vi "Interface_AddImplementVI.vi"(0 "Application":refnum<vi>, 1 "ClassRefToActOn":refnum<vi>, 2 "RefNameInClass":string, 3 "SubInterfaceImplementVI":path, 5 "error in":errorcluster) -> (19 "error out":errorcluster)   [LabVIEW 2012]
uses:
  <vilib>/Utility/miscctls.llb/LVPositionTypeDef.ctl
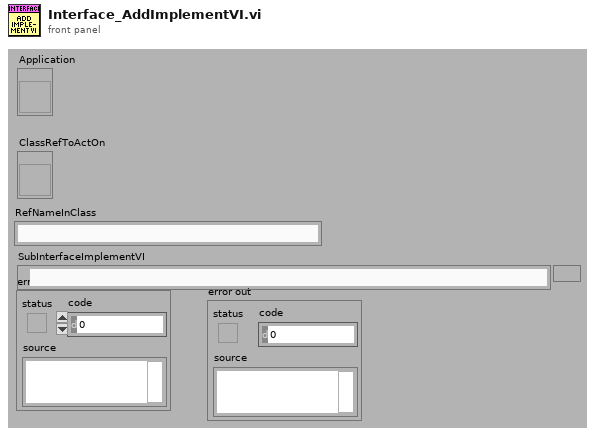
[diagram p1: front panel]
types:
  T1 = typedef "LVPositionTypeDef.ctl" = cluster{"Left":i32, "Top":i32}
  T2 = cluster{"IndTerm":refnum<vi>, "Bundler":refnum<vi>, "SourceTerm":refnum<vi>, "IndOwner":refnum<vi>, "IndPosition":T1, "ViRef":refnum<vi>, "Ind":refnum<vi>, "BundlerInTerm":refnum<vi>, "SourcePosition":T1, "BundlerIndex":i32}
  T3 = typedef "LVRectTypeDef.ctl" = cluster{"Left":i16, "Top":i16, "Right":i16, "Bottom":i16}
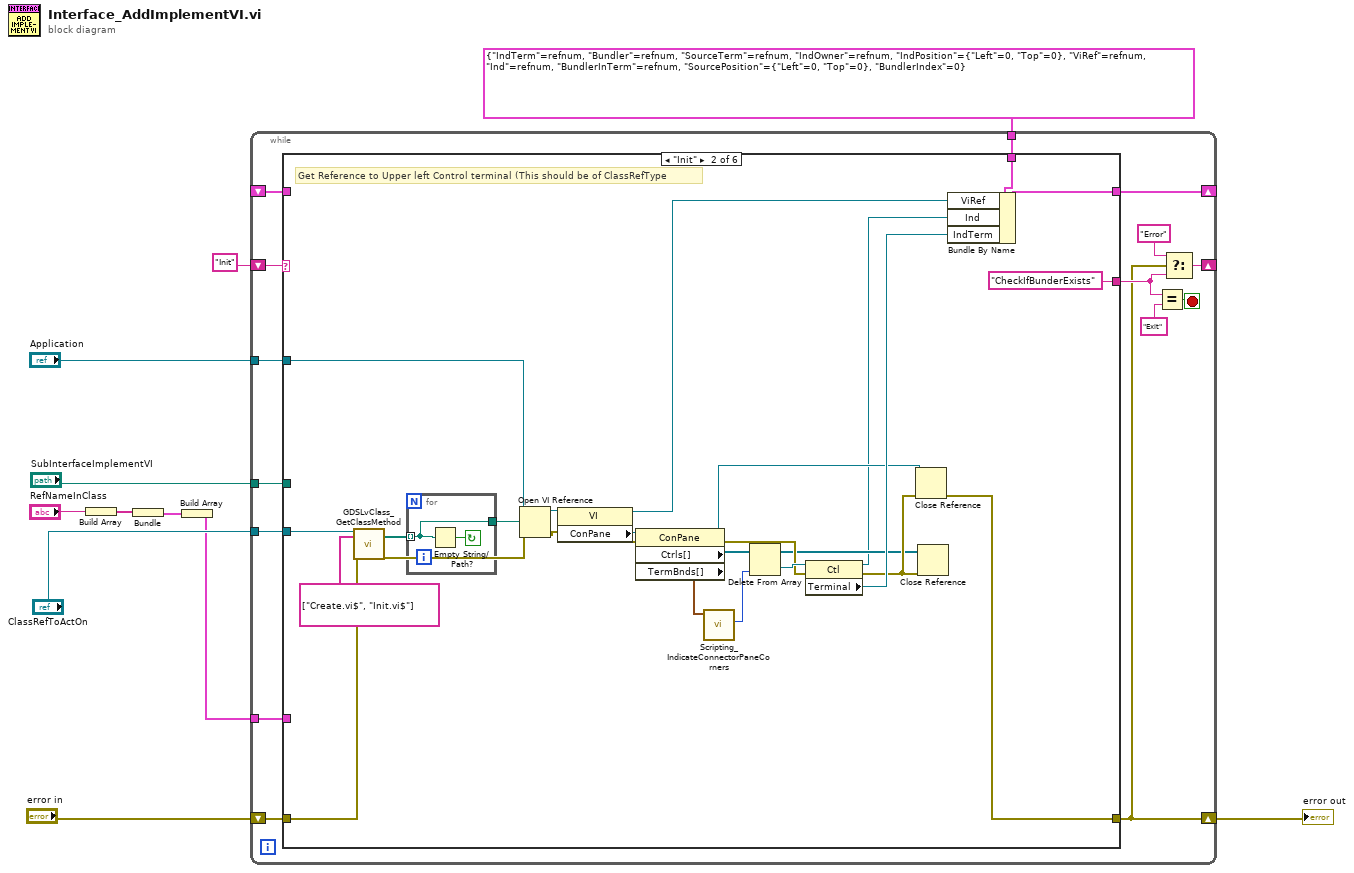
[diagram p0: block diagram]
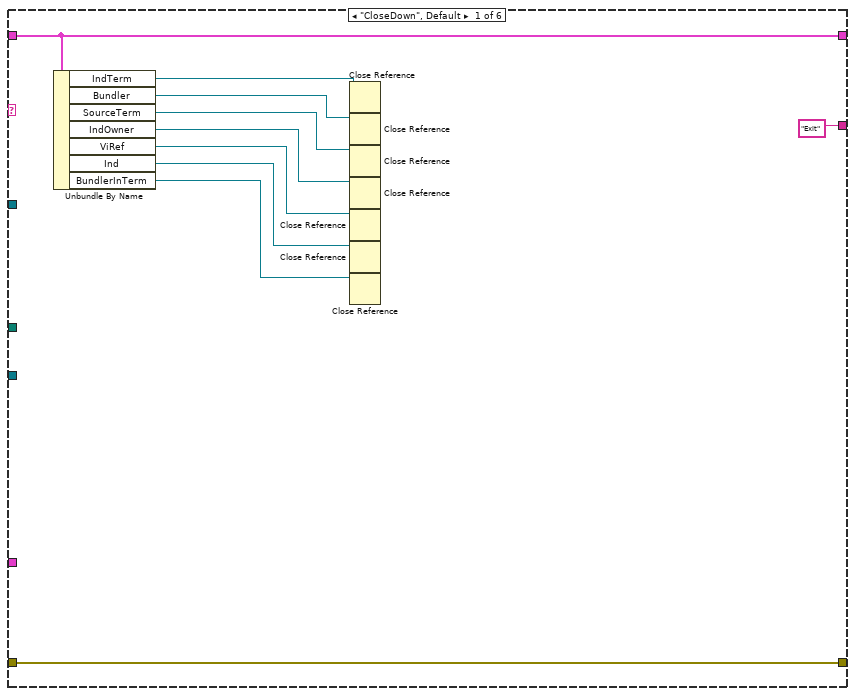
[diagram p2: hidden frame]
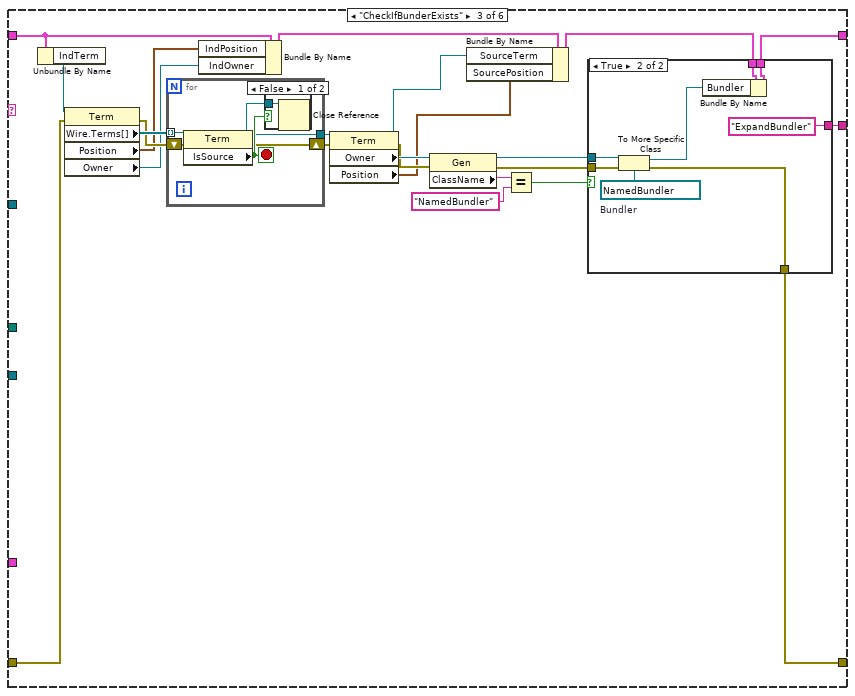
[diagram p3: hidden frame]
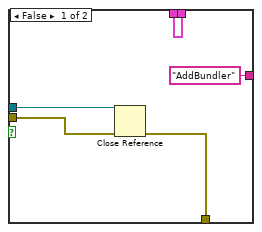
[diagram p4: hidden frame]
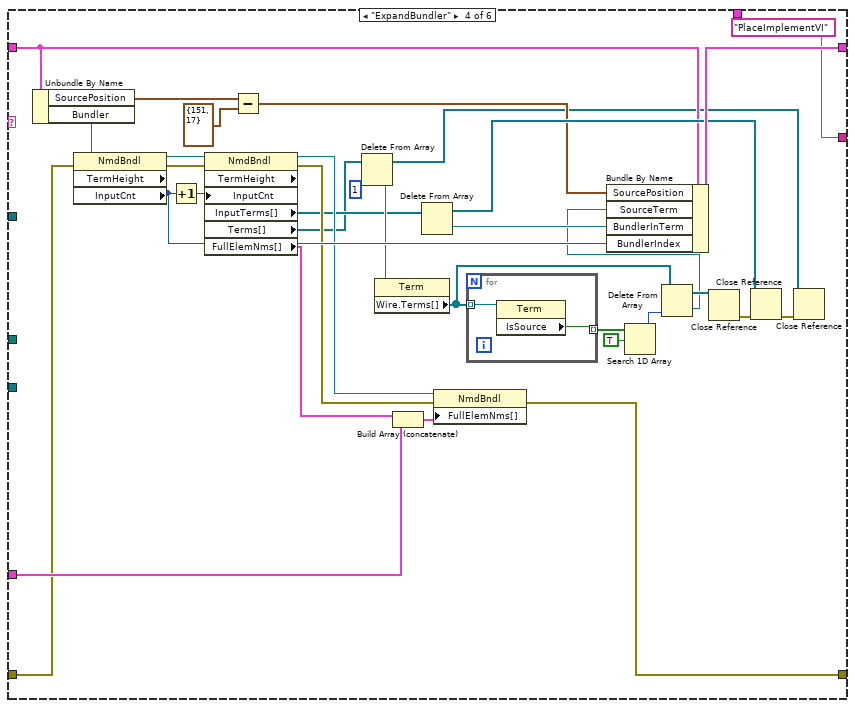
[diagram p6: hidden frame]
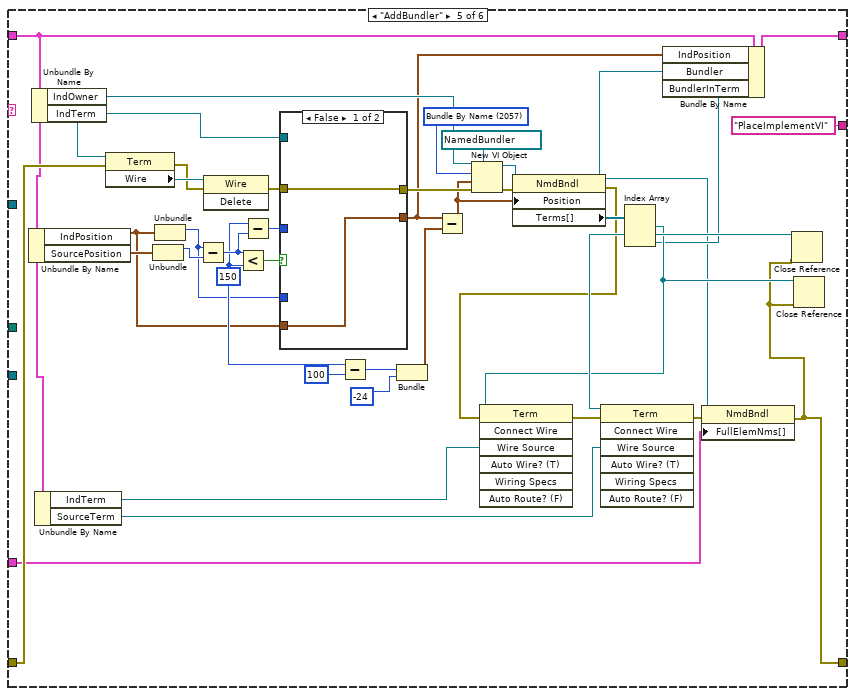
[diagram p7: hidden frame]
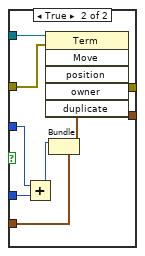
[diagram p8: hidden frame]
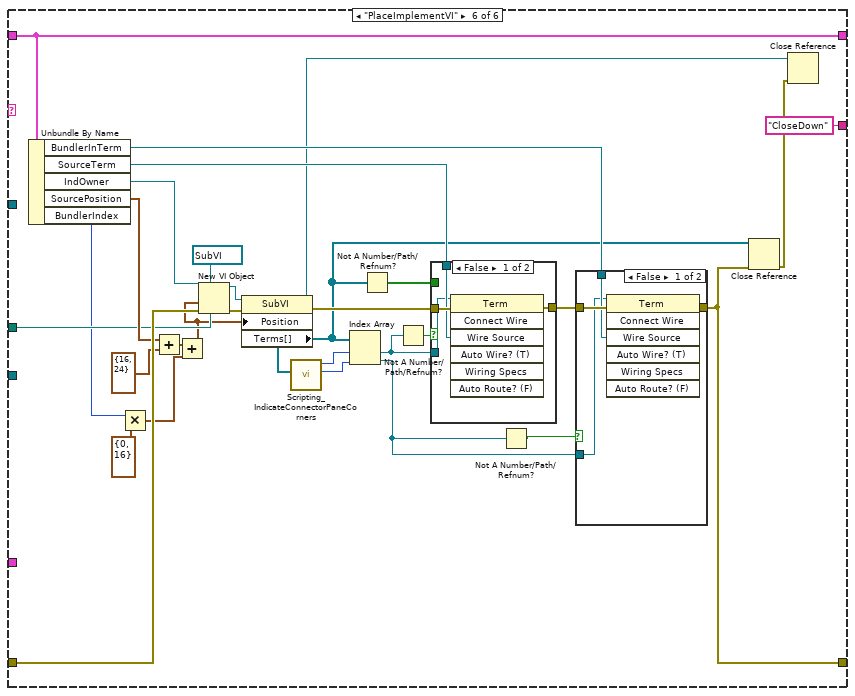
[diagram p9: hidden frame]
diagram:
  n1 = Build Array("RefNameInClass") -> (w4:string[])
  n2 = Bundle(w4) -> (w3:cluster{string[]})  [unwired: 1 in]
  n3 = Build Array(w3) -> (w2:cluster{string[]}[])
  n4 = while {
    shift-right: [w19] -> w8
    shift-left: "error in" -> [w26]
    shift-right: [w24] -> _
    shift-left: "Init" -> [w25]
    shift-right: [w18] -> _
    shift-left: _ -> [w17]
    tunnel: T2 {"IndTerm"=refnum, "Bundler"=refnum, "SourceTerm"=refnum, "IndOwner"=refnum, "IndPosition"={"Left"=0, "Top"=0}, "ViRef"=refnum, "Ind"=refnum, "BundlerInTerm"=refnum, "SourcePosition"={"Left"=0, "Top"=0}, "BundlerIndex"=0} -> [w16]
    tunnel: "ClassRefToActOn" -> [w15]
    tunnel: "Application" -> [w14]
    tunnel: w2 -> [w13]
    tunnel: "SubInterfaceImplementVI" -> [w12]
    stop <- w23 stop-if-true
    n5 = case shown="\"Init\"" w25 {
      tunnel: w26 -> [w36 w44 w70 w127 w179 w218]
      tunnel: [w36 w41 w69 w128 w146 w207] -> w19
      tunnel: ["Exit" "CheckIfBunderExists" w87 "PlaceImplementVI" "PlaceImplementVI" "CloseDown"] -> w20
      tunnel: [w34 w61 w80 w133 w160 w200] -> w18
      tunnel: w17 -> [w34 _ w73 w114 w157 w200]
      tunnel: w16 -> [_ w60 _ _ _ _]
      tunnel: w15 -> [_ w59 _ _ _ _]
      tunnel: w14 -> [_ w55 _ _ _ _]
      tunnel: w13 -> [_ _ _ w129 w145 _]
      tunnel: w12 -> [_ _ _ _ _ w214]
      frame "CloseDown", Default {
        n6 = Unbundle By Name(w34) -> ("IndTerm"=w33:refnum<vi>, "Bundler"=w32:refnum<vi>, "SourceTerm"=w31:refnum<vi>, "IndOwner"=w30:refnum<vi>, "ViRef"=w29:refnum<vi>, "Ind"=w28:refnum<vi>, "BundlerInTerm"=w27:refnum<vi>)
        n7 = Close Reference(reference=w33) -> ()  [unwired: 1 in, 1 out]
        n8 = Close Reference(reference=w32) -> ()  [unwired: 1 in, 1 out]
        n9 = Close Reference(reference=w31) -> ()  [unwired: 1 in, 1 out]
        n10 = Close Reference(reference=w30) -> ()  [unwired: 1 in, 1 out]
        n11 = Close Reference(reference=w29) -> ()  [unwired: 1 in, 1 out]
        n12 = Close Reference(reference=w28) -> ()  [unwired: 1 in, 1 out]
        n13 = Close Reference(reference=w27) -> ()  [unwired: 1 in, 1 out]
      }
      frame "Init" {
        # "Get Reference to Upper left Control terminal (This should be of ClassRefType"
        n14 = call <resource>:"GDSLvClass_GetClassMethod.vi"("Class Refnum In"=w59, "VINames"=string[] ["Create.vi$", "Init.vi$"], "error in (no error)"=w44) -> ("ViPaths"=w57:path[], "error out"=w54:errorcluster)  [unwired: 13 in, 2 out]
        n15 = for {
          tunnel: w57 -> [w63] mode=indexing
          tunnel: [w63] -> w56
          stop <- w64 continue-if-true
          n16 = Empty String/Path?(string/path=w63) -> (empty?=w64:bool)
        }
        n17 = Open VI Reference(application reference (local)=w55, vi path=w56, error in (no error)=w54) -> (vi reference=w53:refnum<vi>, error out=w49:errorcluster)  [unwired: 3 in]
        n18 = property class="VI"(reference=w53, error in=w49) -> (reference out=w43:refnum<vi>, error out=w50:errorcluster, "ConPane"=w52:refnum<vi>)
        n19 = property class="ConPane"(reference=w52, error in=w50) -> (reference out=w42:refnum<vi>, error out=w46:errorcluster, "Ctrls[]"=w45:refnum<vi>[], "TermBnds[]"=w51:T3[])
        n20 = call <resource>:"Scripting_IndicateConnectorPaneCorners.vi"("TermBnds[]"=w51) -> ("RightTop"=w37:i32)  [unwired: 7 in, 3 out]
        n21 = Delete From Array(array=w45, index=w37) -> (deleted portion=w48:refnum<vi>, array with subset deleted=w39:refnum<vi>[])  [unwired: 1 in]
        n22 = property class="Ctl"(reference=w48, error in=w46) -> (reference out=w38:refnum<vi>, error out=w40:errorcluster, "Terminal"=w47:refnum<vi>)
        n23 = Close Reference(reference=w42, error in (no error)=w40) -> (error out=w41:errorcluster)
        n24 = Close Reference(reference=w39, error in (no error)=w40) -> ()  [unwired: 1 out]
        n25 = Bundle By Name(cluster=w60, "ViRef"=w43, "Ind"=w38, "IndTerm"=w47) -> (w61:T2)
      }
      frame "CheckIfBunderExists" {
        n26 = Unbundle By Name(w73) -> ("IndTerm"=w86:refnum<vi>)
        n27 = property class="Term"(reference=w86, error in=w70) -> (error out=w74:errorcluster, "Wire.Terms[]"=w85:refnum<vi>[], "Position"=w72:T1, "Owner"=w71:refnum<vi>)  [unwired: 1 out]
        n28 = for {
          tunnel: w85 -> [w105] mode=indexing
          tunnel: [w103] -> w84
          shift-right: [w102] -> w75
          shift-left: w74 -> [w101]
          stop <- w104 stop-if-true
          n29 = property class="Term"(reference=w105, error in=w101) -> (reference out=w103:refnum<vi>, error out=w102:errorcluster, "IsSource"=w104:bool)
          n30 = case shown="False" w104 {
            tunnel: w103 -> [w106 _]
            frame False {
              n31 = Close Reference(reference=w106) -> ()  [unwired: 1 in, 1 out]
            }
            frame True {
            }
          }
        }
        n32 = Bundle By Name(cluster=w73, "IndPosition"=w72, "IndOwner"=w71) -> (w67:T2)
        n33 = property class="Term"(reference=w84, error in=w75) -> (reference out=w65:refnum<vi>, error out=w76:errorcluster, "Owner"=w83:refnum<vi>, "Position"=w68:T1)
        n34 = property class="Gen"(reference=w83, error in=w76) -> (reference out=w78:refnum<vi>, error out=w77:errorcluster, "ClassName"=w82:string)
        n35 = Bundle By Name(cluster=w67, "SourceTerm"=w65, "SourcePosition"=w68) -> (w66:T2)
        n36 = Equal?(x=w82, y="NamedBundler") -> (x = y?=w79:bool)
        n37 = case shown="True" w79 {
          tunnel: ["AddBundler" "ExpandBundler"] -> w87
          tunnel: w66 -> [w88 w99]
          tunnel: [w88 w98] -> w80
          tunnel: w78 -> [w92 w96]
          tunnel: w77 -> [w89 w95]
          tunnel: [w90 w93] -> w69
          frame False {
            n38 = Close Reference(reference=w92, error in (no error)=w89) -> (error out=w90:errorcluster)
          }
          frame True {
            w97 = refnum<vi> refnum  # Bundler
            n39 = To More Specific Class(target class=w97, reference=w96, error in=w95) -> (specific class reference=w94:refnum<vi>, error out=w93:errorcluster)
            n40 = Bundle By Name(cluster=w99, "Bundler"=w94) -> (w98:T2)
          }
        }
      }
      frame "ExpandBundler" {
        n41 = Unbundle By Name(w114) -> ("SourcePosition"=w113:T1, "Bundler"=w139:refnum<vi>)
        n42 = property class="NmdBndl" props=["TermHeight", "InputCnt"](reference=w139, error in=w127) -> (reference out=w138:refnum<vi>, error out=w137:errorcluster, "InputCnt"=w134:i32)  [unwired: 1 out]
        n43 = Increment(x=w134) -> (x+1=w136:i32)
        n44 = property class="NmdBndl" props=["TermHeight", "InputCnt", "InputTerms[]", "Terms[]", "FullElemNms[]"](reference=w138, error in=w137, "InputCnt"=w136) -> (reference out=w126:refnum<vi>, error out=w132:errorcluster, "InputTerms[]"=w110:refnum<vi>[], "Terms[]"=w109:refnum<vi>[], "FullElemNms[]"=w131:cluster{string[]}[])  [unwired: 1 out]
        n45 = Subtract(x=w113, y=T1 {"Left"=151, "Top"=17}) -> (x-y=w111:T1)
        n46 = Delete From Array(array=w109, index=1) -> (deleted portion=w124:refnum<vi>, array with subset deleted=w107:refnum<vi>[])  [unwired: 1 in]
        n47 = property class="Term"(reference=w124) -> ("Wire.Terms[]"=w121:refnum<vi>[])  [unwired: 1 in, 2 out]
        n48 = Build Array (concatenate)(w131, w129) -> (w130:cluster{string[]}[])
        n49 = Delete From Array(array=w110) -> (deleted portion=w135:refnum<vi>, array with subset deleted=w117:refnum<vi>[])  [unwired: 2 in]
        n50 = property class="NmdBndl"(reference=w126, error in=w132, "FullElemNms[]"=w130) -> (error out=w128:errorcluster)  [unwired: 1 out]
        n51 = for {
          tunnel: w121 -> [w141] mode=indexing
          tunnel: [w140] -> w123 mode=indexing
          n52 = property class="Term"(reference=w141) -> ("IsSource"=w140:bool)  [unwired: 1 in, 2 out]
        }
        n53 = Search 1D Array(1D array=w123, element=TRUE) -> (index of element=w120:i32)  [unwired: 1 in]
        n54 = Delete From Array(array=w121, index=w120) -> (deleted portion=w116:refnum<vi>, array with subset deleted=w119:refnum<vi>[])  [unwired: 1 in]
        n55 = Bundle By Name(cluster=w114, "SourcePosition"=w111, "SourceTerm"=w116, "BundlerInTerm"=w135, "BundlerIndex"=w134) -> (w133:T2)
        n56 = Close Reference(reference=w119) -> (error out=w118:errorcluster)  [unwired: 1 in]
        n57 = Close Reference(reference=w117, error in (no error)=w118) -> (error out=w108:errorcluster)
        n58 = Close Reference(reference=w107, error in (no error)=w108) -> ()  [unwired: 1 out]
      }
      frame "AddBundler" {
        w165 = 2057 items=[".NET Container"=2125, ".NET Refnum"=3441, "2D Picture"=3508, "3D Picture"=23776, "Absolute Value"=1054, "Access Rights"=1412, "ActiveX Container"=2072, "Add"=3915, "Add 1"=1050, "Add Array Elements"=1903, "Agitator"=3831, "AllSpoll"=1960, "Always Copy"=2400, "And"=1061, "And Array Elements"=1911, "Append True/False String"=1511, "Application Refnum"=3412, "Array"=21608, "Array 1"=3300, "Array Constant"=2070, "Array Interface Control"=23777, "Array Max & Min"=1907, "Array Size"=1809, "Array Subset"=2044, "Array To Cluster"=1168, "Array To Spreadsheet String"=1540, "Array of Strings to Path"=1422, "Atmospheric Tank"=3070, "Atmospheric Tank 1"=21751, "Automation Close"=8001, "Automation Open"=8000, "Automation Refnum"=3410, "Avogadro Constant (1/mol)"=23520, "Base 10 Logarithm Of e"=23512, "Bin"=3073, "Bin 1"=21755, "Bitpack to Array"=3135, "Blocking Variable Read"=23786, "Blocking Variable Write"=23789, "Bluetooth Close Connection"=9148, "Bluetooth Create Listener"=9151, "Bluetooth Discover"=9152, "Bluetooth Network Connection Refnum"=3468, "Bluetooth Open Connection"=9153, "Bluetooth Read"=9149, "Bluetooth Wait On Listener"=9147, "Bluetooth Write"=9150, "Boolean Array To Number"=1815, "Boolean To (0,1)"=1167, "Build Array"=2041, "Build Cluster Array"=2047, "Build Matrix"=8500, "Build Path"=1419, "Build Waveform"=2066, "Bundle"=2049, "Bundle By Name"=2057, "Byte Array To String"=1609, "Byte Stream File Refnum"=3408, "CAN Channel"=21966, "CAN Channel 1"=3340, "CAN Channel 2"=2124, "CAN Channel 3"=21817, "CAN Interface"=3339, "CAN Interface 1"=21815, "CAN Interface 2"=2123, "CAN Interface 3"=21964, "CAN Task"=3470, "CAN Task 1"=3471, "CAN Task 2"=21963, "CAN Task 3"=21789, "CPU Information"=24130, "Call By Reference Node"=3901, "Call Chain"=1999, "Call Library Function Node"=2062, "Call Parent Method"=2354, "Cancel Button"=21739, "Cancel Notification"=9107, "Carriage Return Constant"=23500, "Case Structure"=2001, "Cast Unit Bases"=1079, "Check Valve"=3833, "Checkbox"=3117, "Class Specifier Constant"=2094, "Classic Radio Buttons"=22003, "Clear Fixed-Point Overflow Status"=5562, "Close File"=1405, "Close File 1"=8052, "Close Reference"=8011, "Close Variable Connection"=23783, "Cluster"=3400, "Cluster 1"=21607, "Cluster Constant"=2071, "Cluster To Array"=1169, "Code Interface Node"=2050, "Coerce To Type"=2402, "Color Box"=3013, "Color Box Constant"=2120, "Color Box Thin Border"=2905, "Color Ramp"=3022, "Combo Box"=21604, "Combo Box 1"=3304, "Combo Box Constant"=2088, "Complex Conjugate"=1048, "Complex To Polar"=1045, "Complex To Re/Im"=1044, "Compound Arithmetic"=2200, "Compressor"=3832, "Concatenate Strings"=2040, "Conditional Disable Structure"=2064, "Constructor Node"=3904, "Control & Simulation Loop"=2099, "Control Help Window"=1353, "Control Online Help"=1355, "Control Refnum"=3419, "Convert Unit"=2059, "Conveyer"=3827, "Copy"=1416, "Copy 1"=8053, "Cosecant"=1204, "Cosine"=1201, "Cotangent"=1205, "Create Folder"=8055, "Create User Event"=2073, "Current Processor ID"=24131, "Current VI's Menubar"=9000, "Current VI's Path"=1426, "DAQmx Analog Trigger Source"=3336, "DAQmx Analog Trigger Source 1"=2119, "DAQmx Analog Trigger Source 2"=21951, "DAQmx Analog Trigger Source 3"=21774, "DAQmx Device Name"=21773, "DAQmx Device Name 1"=21950, "DAQmx Device Name 2"=2093, "DAQmx Device Name 3"=3318, "DAQmx Global Channel"=3443, "DAQmx Global Channel 1"=21770, "DAQmx Global Channel 2"=21957, "DAQmx Global Channel 3"=3430, "DAQmx Physical Channel"=3335, "DAQmx Physical Channel 1"=21954, "DAQmx Physical Channel 2"=2118, "DAQmx Physical Channel 3"=21777, "DAQmx Scale Name"=21952, "DAQmx Scale Name 1"=21775, "DAQmx Scale Name 2"=3317, "DAQmx Scale Name 3"=2116, "DAQmx Switch"=21953, "DAQmx Switch 1"=3337, "DAQmx Switch 2"=2121, "DAQmx Switch 3"=21776, "DAQmx Task Name"=3442, "DAQmx Task Name 1"=3434, "DAQmx Task Name 2"=21959, "DAQmx Task Name 3"=21778, "DAQmx Terminal"=21955, "DAQmx Terminal 1"=2117, "DAQmx Terminal 2"=21781, "DAQmx Terminal 3"=3319, "Data Cache Size"=24132, "Data Log File Refnum"=3402, "DataSocket Close"=1085, "DataSocket Open"=1084, "DataSocket Read"=1086, "DataSocket Refnum"=3417, "DataSocket Write"=1087, "Date/Time To Seconds"=1308, "Decimal Digit?"=1119, "Decimal String To Number"=1184, "Decimate 1D Array"=2046, "DecomposeArray"=2412, "DecomposeLockDataValRef"=2406, "DecomposeVariant"=2404, "Decrement"=1058, "Default Directory"=1427, "Delete"=8056, "Delete 1"=1417, "Delete Data Value Reference"=2409, "Delete From Array"=3912, "Delete Menu Items"=9004, "Delete Variant Attribute"=8206, "Delete Waveform Attribute"=8209, "Deny Access"=8057, "Dequeue Element"=9113, "Destroy User Event"=2075, "DevClear"=1961, "DevClearList"=1962, "Device Control/Status"=1433, "Device Refnum"=3405, "Diagram Disable Structure"=2054, "Dial"=3050, "Dial 1"=21732, "Digital Data"=3210, "Digital Data 1"=21216, "Digital Waveform Graph"=21718, "Digital Waveform Graph 1"=3511, "Direct Variable Read"=23785, "Direct Variable Write"=23788, "Divide"=1053, "Divide 1"=3918, "Dlg CheckBox"=21924, "Dlg Horiz Scrollbar"=21905, "Dlg Numeric"=2100, "Dlg Numeric 2"=3006, "Dlg String"=2110, "Dlg Vert Scrollbar"=21906, "Down Arrow"=3824, "Down Bow Valve"=3707, "Down Bow Valve 1"=21767, "Down Bow Valve 2"=3807, "Down Rect Valve"=21766, "Down Rect Valve 1"=3706, "Down Rect Valve 2"=3806, "Down Tee"=3818, "Down Tee 1"=3718, "EOF"=1410, "Elementary Charge (C)"=23517, "Empty Array?"=23063, "Empty Path Constant"=23523, "Empty String Constant"=23503, "Empty String/Path?"=1112, "Enable Menu Tracking"=9002, "EnableLocal"=1963, "EnableRemote"=1964, "End of Line Constant"=23525, "Enqueue Element"=9111, "Enqueue Element At Opposite End"=9129, "Enum"=3023, "Enum 1"=21605, "Enum Constant"=2090, "Equal To 0?"=1113, "Equal?"=1102, "Error Ring Constant"=2039, "Event Callback Refnum"=3435, "Event Data Node"=2102, "Event Structure"=2052, "Exchanger"=3828, "Exclusive Or"=1063, "Exponential"=1211, "Exponential (Arg) -1"=1222, "Expression Node"=2201, "FIFO Refnum"=3474, "False Constant"=2006, "Feedback Node, Feedback Node 1"=2353, "FieldPoint IO Point"=21784, "FieldPoint IO Point 1"=3440, "FieldPoint IO Point 2"=3439, "File Dialog"=8058, "File Dialog 1"=8081, "File Path Control"=21730, "File Path Control 1"=3203, "File Path Indicator"=21731, "File Path Indicator 1"=3204, "File/Directory Info"=1413, "File/Directory Info 1"=8082, "FindLstn"=1965, "FindRQS"=1966, "First Call?"=1083, "Fixed-Point Overflow?"=5565, "Fixed-Point to Integer Cast"=5566, "Flat Box"=3602, "Flat Circle"=3605, "Flat Down Triangle"=3623, "Flat Frame"=3608, "Flat Left Triangle"=3620, "Flat Right Triangle"=3621, "Flat Round Button"=3102, "Flat Rounded Box"=3611, "Flat Sequence Structure"=2069, "Flat Square Button"=3103, "Flat Up Triangle"=3622, "Flatten To String"=1164, "Flatten To XML"=8400, "Flattened String To Variant"=8202, "Floating Point Equal?"=23064, "Flush File"=8059, "Flush File 1"=1406, "Flush Queue"=9114, "For Loop"=2002, "Fork"=2194, "Format Date/Time String"=8100, "Format Into File"=2083, "Format Into String"=2081, "Format Value"=1512, "Formula Node"=2004, "Fract/Exp String To Number"=1187, "Framed Color Box"=21019, "Framed Color Box 1"=3008, "Free Label"=2321, "Furnace"=3829, "GPIB Clear"=1954, "GPIB Initialization"=1957, "GPIB Misc"=1956, "GPIB Read"=1951, "GPIB Serial Poll"=1955, "GPIB Status"=1959, "GPIB Trigger"=1953, "GPIB Wait"=1958, "GPIB Write"=1950, "Gauge"=21009, "Gauge 1"=3040, "Generate Front Panel Activity"=1329, "Generate Occurrence"=1700, "Generate User Event"=2074, "Generate User-Defined Trace Event"=2250, "Get Datalog Position"=8061, "Get Date/Time In Seconds"=1303, "Get Date/Time String"=1600, "Get Drag Drop Data"=9154, "Get File Position"=8062, "Get File Size"=8063, "Get Fixed-Point Components"=11163, "Get Help Window Status"=1354, "Get Matrix Diagonal"=8501, "Get Matrix Elements"=8502, "Get Menu Item Info"=9005, "Get Menu Selection"=9001, "Get Menu Short Cut Info"=9007, "Get Notifier Status"=9103, "Get Number of Records"=8064, "Get Permissions"=8065, "Get Queue Status"=9110, "Get Submatrix"=8503, "Get Type and Creator"=8066, "Get Variant Attribute"=8205, "Get Volume Info"=8067, "Get Waveform Attribute"=8208, "Get Waveform Components"=2067, "Global Variable"=2060, "Gravitational Constant (N m2/kg2)"=23519, "Greater Or Equal To 0?"=1114, "Greater Or Equal?"=1103, "Greater Than 0?"=1117, "Greater?"=1110, "Handle Peek"=1604, "Handle Poke"=1605, "Hex Digit?"=1123, "Hexadecimal String To Number"=1185, "Hopper"=21754, "Hopper 1"=3072, "Horiz Line"=3821, "Horiz Pipe"=3710, "Horiz Pipe 1"=3810, "Horizontal Button Box"=3636, "Horizontal Fill Slide"=3012, "Horizontal Fill Slide 1"=21100, "Horizontal Graduated Bar"=21106, "Horizontal Pointer Slide"=21101, "Horizontal Pointer Slide 1"=3011, "Horizontal Progress Bar"=21102, "Horizontal Scrollbar"=21110, "Horizontal Slide"=3010, "Horizontal Slide Switch"=3114, "Horizontal Smooth Box"=3633, "Horizontal Splitter Bar"=21861, "Horizontal Splitter Bar (Classic)"=21863, "Horizontal Splitter Bar (System)"=21865, "Horizontal Switch"=3108, "Horizontal Tank"=3071, "Horizontal Toggle Switch"=3110, "Horizontal Toggle Switch 1"=21700, "Hyperbolic Cosecant"=23053, "Hyperbolic Cosine"=1215, "Hyperbolic Cotangent"=23055, "Hyperbolic Secant"=23054, "Hyperbolic Sine"=1214, "Hyperbolic Tangent"=1216, "IMAQ Session"=3415, "IP To String"=1710, "IVI Delete Session"=8103, "IVI Logical Name"=3420, "IVI Logical Name 1"=3414, "IVI Logical Name 2"=21736, "IVI New Session"=8102, "Implies"=1080, "In Place Element Structure"=2360, "In Range and Coerce"=1127, "Include Fixed-Point Overflow Status"=5564, "Increment"=1057, "Index & Bundle Cluster Array"=2056, "Index Array"=2042, "Index String Array"=1531, "Initialize Array"=2053, "Inline C Node"=2104, "Insert Into Array"=3911, "Insert Menu Items"=9003, "Integer to Fixed-Point Cast"=5567, "Intensity Chart"=21719, "Intensity Chart 1"=3509, "Intensity Graph"=21720, "Intensity Graph 1"=3510, "Interleave 1D Arrays"=2045, "Interpolate 1D Array"=1905, "Inverse Cosecant"=23050, "Inverse Cosine"=1207, "Inverse Cotangent"=23052, "Inverse Hyperbolic Cosecant"=23056, "Inverse Hyperbolic Cosine"=1218, "Inverse Hyperbolic Cotangent"=23058, "Inverse Hyperbolic Secant"=23057, "Inverse Hyperbolic Sine"=1217, "Inverse Hyperbolic Tangent"=1219, "Inverse Secant"=23051, "Inverse Sine"=1206, "Inverse Tangent"=1208, "Inverse Tangent (2 Input)"=1228, "Invoke Node"=3900, "IrDA Close Connection"=9144, "IrDA Create Listener"=9140, "IrDA Discover"=9141, "IrDA Network Connection Refnum"=3450, "IrDA Open Connection"=9142, "IrDA Read"=9145, "IrDA Wait On Listener"=9143, "IrDA Write"=9146, "Join"=2195, "Join Numbers"=1171, "Junction"=2197, "Knob"=21000, "Knob 1"=3005, "LED Button"=3116, "LabVIEW Object"=3457, "Label"=21960, "Labeled Oblong Button"=3125, "Labeled Rectangular Button"=3124, "Labeled Round Button"=3122, "Labeled Square Button"=3123, "Leak Variant Value Reference"=2410, "Left Arrow"=3826, "Left Bow Valve"=3701, "Left Bow Valve 1"=3801, "Left Bow Valve 2"=21761, "Left Down Elbow"=3711, "Left Down Elbow 1"=3811, "Left Pump"=3713, "Left Pump 1"=3813, "Left Rect Valve"=3700, "Left Rect Valve 1"=21760, "Left Rect Valve 2"=3800, "Left Tee"=3709, "Left Tee 1"=3809, "Left Up Elbow"=3808, "Left Up Elbow 1"=3708, "Less Or Equal To 0?"=1115, "Less Or Equal?"=1104, "Less Than 0?"=1118, "Less?"=1111, "Lexical Class"=1126, "Line Feed Constant"=23501, "List Directory"=1418, "List Folder"=8083, "Listbox"=21792, "Listbox 1"=21806, "Listbox Symbol Ring Constant"=2038, "Local Variable"=2061, "Lock Range"=1411, "Logarithm Base 10"=1210, "Logarithm Base 2"=1225, "Logarithm Base X"=1224, "Logical Shift"=1081, "Lossy Enqueue Element"=9130, "Lowered Rounded Box"=3638, "MATLAB script"=9020, "Machine Epsilon"=23528, "MakeAddr"=1967, "Mantissa & Exponent"=1150, "Match First String"=1532, "Match Pattern"=1535, "Match True/False String"=1533, "MathScript Call By Reference Node"=3906, "MathScript Node"=2357, "Matrix Size"=8507, "Max & Min"=1108, "Menu Refnum"=3413, "Menu Ring"=3018, "Menu Ring 1"=21600, "Menu-Popup Ring"=3017, "Merge Signals"=2350, "Meter"=21008, "Meter 1"=3030, "Mixed Signal Graph"=21721, "Molar Gas Constant (J/(mol K))"=23522, "Motion Resource"=21787, "Motion Resource 1"=3448, "Motion Resource 2"=3449, "Motor"=3720, "Motor 1"=3820, "Move"=1415, "Move 1"=8068, "Multi-Segment Pipe"=23780, "Multicolumn Listbox"=21799, "Multicolumn Listbox 1"=21791, "Multiple Selection Listbox"=3208, "Multiply"=1052, "Multiply 1"=3917, "Multiply Array Elements"=1904, "Multirate Structure"=2199, "Natural Logarithm"=1209, "Natural Logarithm (Arg +1)"=1221, "Natural Logarithm Base"=23510, "Natural Logarithm Of 10"=23513, "Natural Logarithm Of 2"=23514, "Natural Logarithm Of Pi"=23508, "Negate"=1069, "Negative Infinity"=23509, "New Data Value Reference"=2408, "New Directory"=1402, "New File"=1404, "New VI"=8014, "New VI Object"=8015, "Not"=1064, "Not A Number/Path/Refnum?"=1128, "Not A Path Constant"=23524, "Not And"=1071, "Not Equal To 0?"=1116, "Not Equal?"=1105, "Not Exclusive Or"=1073, "Not Or"=1072, "Not a Refnum Constant"=23526, "Not a Shared Variable"=23527, "Notifier Refnum"=3423, "Number To Boolean Array"=1814, "Number To Decimal String"=1180, "Number To Engineering String"=1183, "Number To Exponential String"=1505, "Number To Fractional String"=1506, "Number To Hexadecimal String"=1181, "Number To Octal String"=1182, "Number of Cache Levels"=24133, "Numeric Constant"=2005, "Numeric Control"=3000, "Numeric Control 1"=21003, "Numeric Indicator"=3001, "Numeric Indicator 1"=21004, "OK Button"=21738, "OLE Variant"=3150, "Obtain Notifier"=9101, "Obtain Queue"=9108, "Occurrence Refnum"=3406, "Octal Digit?"=1129, "Octal String To Number"=1186, "Old VISA Open"=1921, "One Button Dialog"=1340, "Open Application Reference"=8012, "Open Device"=1430, "Open File"=1403, "Open Tank"=21752, "Open Tank 1"=3074, "Open VI Object Reference"=8013, "Open VI Reference"=8010, "Open Variable Connection"=23779, "Open Variable Connection in Background"=23791, "Open and Verify Variable Connection"=23790, "Open/Create/Replace Datalog"=8054, "Open/Create/Replace File"=8050, "Or"=1062, "Or Array Elements"=1910, "PPoll"=1969, "PPollConfig"=1970, "PPollUnconfig"=1971, "Package Matrix"=23001, "PassControl"=1968, "Path Constant"=2009, "Path To String"=1077, "Path Type"=1421, "Path to Array of Strings"=1423, "Pi"=23504, "Pi Divided By 2"=23506, "Pi Multiplied By 2"=23505, "Pick Line"=1510, "Pict Ring"=21602, "Pict Ring 1"=3015, "PixMap"=3505, "PixMap (Do not touch it!!)"=3507, "Planck's Constant (J/Hz)"=23516, "Platform Flat Square Button"=3134, "Plug-In Control"=21820, "Polar To Complex"=1047, "Polar To Re/Im"=23061, "Positive Infinity"=23515, "Power Of 10"=1212, "Power Of 2"=1223, "Power Of X"=1213, "Preserve Run-Time Class"=8018, "Pressure Tank"=3075, "Pressure Tank 1"=21753, "Preview Queue Element"=9112, "Printable?"=1124, "Property Node"=1920, "Pulldown Menu Ring"=3061, "Push Button"=21001, "Queue Refnum"=3424, "Quit LabVIEW"=1352, "Quotient & Remainder"=1056, "RT FIFO Create"=24000, "RT FIFO Delete"=24003, "RT FIFO Read"=24001, "RT FIFO Write"=24002, "Radio Buttons"=22001, "Raised Box"=3600, "Raised Box 1"=3637, "Raised Circle"=3603, "Raised Down Triangle"=3615, "Raised Frame"=3606, "Raised Left Triangle"=3612, "Raised Right Triangle"=3613, "Raised Rounded Box"=3609, "Raised Up Triangle"=3614, "Random Number (0-1)"=1070, "RcvRespMsg"=1972, "Re/Im To Complex"=1046, "Re/Im To Polar"=23060, "Read Datalog"=8069, "Read Device"=1432, "Read File"=1407, "Read Variable"=23781, "Read from Binary File"=8051, "Read from Text File"=8070, "ReadStatus"=1973, "Receive"=1974, "ReceiveSetup"=1975, "Recessed Box"=3601, "Recessed Circle"=3604, "Recessed Down Triangle"=3619, "Recessed Frame"=3607, "Recessed Left Triangle"=3616, "Recessed Menu Ring"=3019, "Recessed Right Triangle"=3617, "Recessed Rounded Box"=3610, "Recessed Up Triangle"=3618, "Reciprocal"=1059, "Reciprocal Of Pi"=23507, "Reciprocal Of e"=23511, "RecomposeArray"=2403, "RecomposeUnlockDataValRef"=2407, "RecomposeVariant"=2405, "Rectangular Stop Button"=3128, "Refnum to Path"=1424, "Refnum to Session"=2306, "Region"=2196, "Register Event Callback"=2078, "Register For Events"=2065, "Register Session"=2319, "Release Notifier"=9102, "Release Queue"=9109, "Remove Fixed-Point Overflow Status"=5563, "Replace Array Subset"=3910, "Replace Substring"=3913, "Request Deallocation"=1610, "ResetSys"=1976, "Reshape Array"=2055, "Resize Matrix"=8508, "Reverse 1D Array"=1900, "Reverse String"=1537, "Right Arrow"=3825, "Right Bow Valve"=21765, "Right Bow Valve 1"=3705, "Right Bow Valve 2"=3805, "Right Down Elbow"=3817, "Right Down Elbow 1"=3717, "Right Pump"=3719, "Right Pump 1"=3819, "Right Rect Valve"=3804, "Right Rect Valve 1"=3704, "Right Rect Valve 2"=21764, "Right Tee"=3715, "Right Tee 1"=3815, "Right Up Elbow"=3814, "Right Up Elbow 1"=3714, "Ring Constant"=2008, "Rocker"=21002, "Rotary Feeder"=3830, "Rotate"=1082, "Rotate 1D Array"=1906, "Rotate Left With Carry"=1606, "Rotate Right With Carry"=1607, "Rotate String"=1536, "Round Button"=3100, "Round LED"=3120, "Round LED 1"=21012, "Round Light"=3104, "Round Push Button"=3112, "Round Push Button 2"=3118, "Round Radio Button"=3106, "Round Stop Button"=3127, "Round To Nearest"=1055, "Round Toward +Infinity"=1076, "Round Toward -Infinity"=1075, "Rydberg Constant (1/m)"=23521, "Scale By Power Of 2"=1074, "Scan From File"=2082, "Scan From String"=2080, "Scan String For Tokens"=8101, "Scan Value"=1534, "Scanned Variable Read"=23784, "Scanned Variable Write"=23787, "Search 1D Array"=1901, "Search and Replace String"=3914, "Search/Split String"=1538, "Secant"=1203, "Seconds To Date/Time"=1309, "Seek"=1409, "Select"=1516, "Send"=1977, "Send Notification"=9104, "SendCmds"=1978, "SendDataBytes"=1979, "SendIFC"=1980, "SendLLO"=1982, "SendList"=1981, "SendSetup"=1983, "Session to Refnum"=2307, "Set Datalog Position"=8072, "Set File Position"=8073, "Set File Size"=8074, "Set Matrix Diagonal"=8504, "Set Matrix Elements"=8505, "Set Menu Item Info"=9006, "Set Number of Records"=8075, "Set Occurrence"=1702, "Set Permissions"=8076, "Set Submatrix"=8506, "Set Type and Creator"=8077, "Set Variant Attribute"=8204, "Set Waveform Attribute"=8207, "SetRWLS"=1984, "SetTimeOut"=1985, "Shared Variable"=23778, "Shared Variable Constant"=3473, "Shared Variable Control"=3472, "Shared Variable Control 1"=21814, "Shared Variable to String"=1831, "Sign"=1049, "Simple Horizontal Slide"=3003, "Simple Numeric"=3029, "Simple Numeric 1"=2900, "Simple String"=2115, "Simple Vertical Slide"=3002, "Sinc"=1227, "Sine"=1200, "Sine & Cosine"=1220, "Size Handle"=1603, "Slide Switch"=21011, "Sort 1D Array"=1120, "Sort Array of String, Sort Array of String 1"=23065, "Speed Of Light In Vacuum (m/sec)"=23518, "Split 1D Array"=1908, "Split Button"=21020, "Split Number"=1170, "Split Signals"=2351, "Spreadsheet String To Array"=1539, "Square"=23059, "Square Button"=3101, "Square LED"=3121, "Square LED 1"=21013, "Square Light"=3105, "Square Push Button"=3113, "Square Push Button 2"=3119, "Square Radio Button"=3107, "Square Root"=1060, "Stacked Sequence Structure"=2000, "State"=2198, "State Diagram"=2051, "Static VI Reference"=2084, "Stop"=1350, "Stop Button"=21230, "String Constant"=2007, "String Control"=3200, "String Control 1"=21701, "String Indicator"=3201, "String Indicator 1"=21702, "String Length"=1502, "String Subset"=1503, "String To Byte Array"=1608, "String To IP"=1711, "String To Path"=1078, "String to Shared Variable"=1830, "Strip Path"=1420, "SubPanel"=21810, "SubPanel (Classic)"=21811, "SubPanel (System)"=21823, "Subtract"=1051, "Subtract 1"=3916, "Swap Bytes"=1162, "Swap Values"=2401, "Swap Vector Element"=1912, "Swap Words"=1163, "System Button"=3130, "System Cancel Button"=3131, "System Checkbox"=3132, "System Chiseled Line"=3632, "System Colored Rectangle"=3625, "System Combo Box"=21917, "System Enum"=3062, "System Horizontal Pointer Slide"=21902, "System Horizontal Progress Bar"=21910, "System Horizontal Slide"=21904, "System Label"=21961, "System Listbox"=21805, "System Mixed Checkbox"=21333, "System Multicolumn Listbox"=21798, "System Numeric"=21919, "System Path Control"=21922, "System Pict Ring"=21925, "System Radio Button"=3133, "System Radio Buttons"=22002, "System Recessed Frame"=3624, "System Ring"=3060, "System Spin Control"=21900, "System String"=21920, "System Tab Control"=3331, "System Table"=21797, "System Time Stamp"=21967, "System Tree"=21794, "System Vertical Pointer Slide"=21901, "System Vertical Progress Bar"=21909, "System Vertical Slide"=21903, "TCP Close Connection"=1713, "TCP Create Listener"=1717, "TCP Flattened Read"=1718, "TCP Flattened Write"=1719, "TCP Flex Read"=1720, "TCP Flex Write"=1721, "TCP Network Connection Refnum"=3407, "TCP Open Connection"=1715, "TCP Read"=1716, "TCP Wait On Listener"=1712, "TCP Write"=1714, "TDMS Close"=24113, "TDMS Defragment"=24119, "TDMS File"=3477, "TDMS Flush"=24117, "TDMS Get Properties"=24115, "TDMS List Contents"=24116, "TDMS Open"=24112, "TDMS Read"=24111, "TDMS Refnum To File ID"=24120, "TDMS Set Properties"=24114, "TDMS Write"=24110, "TDMS Write IP"=24118, "Tab Constant"=23502, "Tab Control"=3330, "Tab Control 1"=3332, "Table"=21796, "Table 1"=21790, "Tag Attribute Ring"=2063, "Tangent"=1202, "Tank"=21006, "Tank 1"=3020, "Temporary Directory"=1435, "TestSRQ"=1986, "TestSys"=1987, "Text & Pict Ring"=21603, "Text & Pict Ring 1"=3016, "Text Button"=21015, "Text Ring"=21601, "Text Ring 1"=3014, "Text to UTF-8"=23066, "Thermometer"=21007, "Thermometer 1"=3021, "Thick Chiseled Line"=3630, "Thick Line"=3629, "Thick Line with Arrow"=3631, "Thick Lowered Box"=3635, "Thin Chiseled Line"=3627, "Thin Line"=3626, "Thin Line with Arrow"=3628, "Threshold 1D Array"=1909, "Tick Count (ms)"=1300, "Time Stamp Constant"=2068, "Time Stamp Control"=21913, "Time Stamp Control 1"=5555, "Time Stamp Indicator"=21914, "Time Stamp Indicator 1"=5556, "Timed Loop"=5570, "Timed Sequence"=5573, "To Byte Integer"=1140, "To Double Precision Complex"=1152, "To Double Precision Float"=1147, "To Extended Precision Complex"=1154, "To Extended Precision Float"=1149, "To Fixed-Point"=5561, "To Long Integer"=1142, "To Lower Case"=1189, "To More Generic Class"=8017, "To More Specific Class"=8016, "To OLE Variant"=8002, "To Probe String"=2413, "To Quad Integer"=1155, "To Single Precision Complex"=1151, "To Single Precision Float"=1146, "To Time Stamp"=5560, "To Unsigned Byte Integer"=1143, "To Unsigned Long Integer"=1145, "To Unsigned Quad Integer"=1156, "To Unsigned Word Integer"=1144, "To Upper Case"=1188, "To Variant"=8201, "To Word Integer"=1141, "Traditional DAQ Channel"=21733, "Traditional DAQ Channel 1"=2085, "Traditional DAQ Channel 2"=3320, "Transpose 1D Array"=23068, "Transpose 2D Array"=1902, "Transpose Matrix"=8509, "Tree"=21819, "Tree 1"=21793, "Trigger"=1988, "TriggerList"=1989, "Two Button Dialog"=1341, "Type Cast"=1166, "Type and Creator"=1434, "UDP Close"=1726, "UDP Multicast Open"=1727, "UDP Network Connection Refnum"=3418, "UDP Open"=1723, "UDP Read"=1724, "UDP Write"=1725, "UTF-8 to Text"=23067, "Unbitpack from Array"=3136, "Unbundle"=2048, "Unbundle By Name"=2058, "Unflatten From String"=1165, "Unflatten From XML"=8401, "Unleak Variant Value Reference"=2411, "Unpackage Matrix"=23000, "Unregister For Events"=2076, "Unregister Session"=2320, "Up Arrow"=3823, "Up Bow Valve"=3703, "Up Bow Valve 1"=3803, "Up Bow Valve 2"=21763, "Up Rect Valve"=3702, "Up Rect Valve 1"=21762, "Up Rect Valve 2"=3802, "Up Tee"=3712, "Up Tee 1"=3812, "User Defined Refnum"=3428, "User Defined Refnum Tag"=21745, "User Defined Refnum Tag 1"=3429, "User Defined Refnum Tag Constant"=3426, "User Defined Refnum Tag Flatten"=21747, "User Defined Refnum Tag Flatten 1"=3454, "User Defined Tag"=21749, "User Defined Tag 1"=3329, "User Defined Tag Constant"=2114, "User Item"=3506, "VI Library"=1425, "VI Refnum"=3422, "VI Server Reference"=2091, "VISA Assert Interrupt Signal"=2309, "VISA Assert Trigger"=1929, "VISA Assert Utility Signal"=2310, "VISA Clear"=1927, "VISA Close"=1922, "VISA Disable Event"=1940, "VISA Discard Events"=1941, "VISA Enable Event"=1942, "VISA Find Resource"=1923, "VISA Flush I/O Buffer"=2302, "VISA GPIB Command"=2315, "VISA GPIB Control ATN"=2316, "VISA GPIB Control REN"=2304, "VISA GPIB Pass Control"=2317, "VISA GPIB Send IFC"=2318, "VISA In 16"=1930, "VISA In 32"=1944, "VISA In 64"=2140, "VISA In 8"=1936, "VISA Lock"=1993, "VISA Map Address"=1932, "VISA Map Trigger"=2311, "VISA Memory Allocation"=1997, "VISA Memory Allocation Ex"=2146, "VISA Memory Free"=1998, "VISA Move"=2303, "VISA Move In 16"=1948, "VISA Move In 32"=1991, "VISA Move In 64"=2144, "VISA Move In 8"=1946, "VISA Move Out 16"=1949, "VISA Move Out 32"=1992, "VISA Move Out 64"=2145, "VISA Move Out 8"=1947, "VISA Open"=2308, "VISA Out 16"=1931, "VISA Out 32"=1945, "VISA Out 64"=2141, "VISA Out 8"=1937, "VISA Peek 16"=1934, "VISA Peek 32"=1995, "VISA Peek 64"=2142, "VISA Peek 8"=1938, "VISA Poke 16"=1935, "VISA Poke 32"=1996, "VISA Poke 64"=2143, "VISA Poke 8"=1939, "VISA Read"=1925, "VISA Read STB"=1928, "VISA Read To File"=2313, "VISA Refnum to Session"=2300, "VISA Resource Name"=3421, "VISA Set I/O Buffer Size"=2301, "VISA Status Description"=1924, "VISA USB Control In"=2086, "VISA USB Control Out"=2087, "VISA Unlock"=1994, "VISA Unmap Address"=1933, "VISA Unmap Trigger"=2312, "VISA VXI Cmd or Query"=2305, "VISA Wait on Event"=1943, "VISA Write"=1926, "VISA Write From File"=2314, "VISA resource name"=3409, "VISA resource name 1"=21737, "Variable Class Specifier Constant"=2106, "Variable Configuration"=3475, "Variant"=3310, "Variant To Data"=8003, "Variant To Flattened String"=8203, "Vert Line"=3822, "Vert Pipe"=3816, "Vert Pipe 1"=3716, "Vert Rocker"=21740, "Vertical Fill Slide"=21014, "Vertical Fill Slide 1"=3009, "Vertical Graduated Bar"=21107, "Vertical Pointer Slide"=21017, "Vertical Pointer Slide 1"=3007, "Vertical Progress Bar"=21104, "Vertical Scrollbar"=21111, "Vertical Slide"=3004, "Vertical Slide Switch"=21741, "Vertical Slide Switch 1"=3115, "Vertical Smooth Box"=3634, "Vertical Splitter Bar"=21860, "Vertical Splitter Bar (Classic)"=21862, "Vertical Splitter Bar (System)"=21864, "Vertical Switch"=3109, "Vertical Toggle Switch"=21005, "Vertical Toggle Switch 1"=3111, "Volume Info"=1414, "Wait (ms)"=1302, "Wait For Activity"=1722, "Wait For Front Panel Activity"=1328, "Wait Until Next ms Multiple"=1327, "Wait for GPIB RQS"=1952, "Wait on Notification"=9105, "Wait on Notification from Multiple"=9106, "Wait on Notification from Multiple with Notifier History"=9132, "Wait on Notification with Notifier History"=9131, "Wait on Occurrence"=1701, "WaitSRQ"=1990, "Waveform Chart"=21010, "Waveform Chart 1"=3501, "Waveform Chart 2"=21717, "Waveform Graph"=21703, "Waveform Graph 1"=3504, "While Loop"=2003, "While Loop 1"=2352, "White Space?"=1125, "Write Datalog"=8079, "Write Device"=1431, "Write File"=1408, "Write Variable"=23782, "Write to Binary File"=8078, "Write to Text File"=8080, "XY Graph"=21716, "XY Graph 1"=3500, "Y-th Root of X"=23062]
        w171 = 150 ("y")
        n59 = Unbundle By Name(w157) -> ("IndPosition"=w142:T1, "SourcePosition"=w177:T1)
        n60 = Unbundle By Name(w157) -> ("IndOwner"=w166:refnum<vi>, "IndTerm"=w153:refnum<vi>)
        n61 = Unbundle By Name(w157) -> ("IndTerm"=w156:refnum<vi>, "SourceTerm"=w155:refnum<vi>)
        n62 = property class="Term"(reference=w153, error in=w179) -> (error out=w180:errorcluster, "Wire"=w181:refnum<vi>)  [unwired: 1 out]
        n63 = Unbundle(w177) -> ("Left"=w152:i32)  [unwired: 1 out]
        n64 = Unbundle(w142) -> ("Left"=w143:i32)  [unwired: 1 out]
        n65 = Subtract(x=w143, y=w152) -> (x-y=w176:i32)
        n66 = invoke class="Wire" method="Delete"(reference=w181, error in=w180) -> (error out=w174:errorcluster)  [unwired: 1 in, 2 out]
        n67 = Less?(x=w176, y=w171) -> (x < y?=w178:bool)
        n68 = Subtract(x=w171, y=w176) -> (x-y=w175:i32)
        n69 = case shown="False" w178 {
          tunnel: w153 -> [_ w191]
          tunnel: w142 -> [w182 w190]
          tunnel: w143 -> [_ w189]
          tunnel: w175 -> [_ w188]
          tunnel: w174 -> [w183 w186]
          tunnel: [w183 w185] -> w172
          tunnel: [w182 w184] -> w144
          frame False {
          }
          frame True {
            n70 = Add(x=w188, y=w189) -> (x+y=w187:i32)
            n71 = Bundle(cluster=w190, "Left"=w187) -> (w184:T1)  [unwired: 1 in]
            n72 = invoke class="Term" method="Move"(reference=w191, error in=w186, "position"=w184) -> (error out=w185:errorcluster)  [unwired: 3 in, 5 out]
          }
        }
        n73 = Subtract(x=w171, y=100) -> (x-y=w169:i32)
        n74 = Bundle(w169, "y"=-24) -> (w167:cluster{i32, "y":i32})  [unwired: 1 in]
        n75 = Subtract(x=w144, y=w167) -> (x-y=w161:T1)
        n76 = New VI Object(vi object class=refnum<vi> refnum ("Bundler"), owner refnum=w166, style=w165, position/next to=w161, 8:w172) -> (object refnum=w162:refnum<vi>, 0:w163:errorcluster)  [unwired: 3 in]
        n77 = property class="NmdBndl"(reference=w162, error in=w163, "Position"=w161) -> (reference out=w147:refnum<vi>, error out=w149:errorcluster, "Terms[]"=w159:refnum<vi>[])
        n78 = Index Array(array=w159) -> (element #1=w151:refnum<vi>, element #2=w154:refnum<vi>, element #3=w150:refnum<vi>)  [unwired: 3 in]
        n79 = invoke class="Term" method="Connect Wire"(reference=w151, error in=w149, "Wire Source"=w156) -> (error out=w158:errorcluster)  [unwired: 4 in, 6 out]
        n80 = invoke class="Term" method="Connect Wire"(reference=w154, error in=w158, "Wire Source"=w155) -> (error out=w148:errorcluster)  [unwired: 4 in, 6 out]
        n81 = Bundle By Name(cluster=w157, "IndPosition"=w144, "Bundler"=w147, "BundlerInTerm"=w150) -> (w160:T2)
        n82 = property class="NmdBndl"(reference=w147, error in=w148, "FullElemNms[]"=w145) -> (error out=w146:errorcluster)  [unwired: 1 out]
        n83 = Close Reference(reference=w154, error in (no error)=w146) -> ()  [unwired: 1 out]
        n84 = Close Reference(reference=w151, error in (no error)=w146) -> ()  [unwired: 1 out]
      }
      frame "PlaceImplementVI" {
        n85 = Unbundle By Name(w200) -> ("BundlerInTerm"=w208:refnum<vi>, "SourceTerm"=w210:refnum<vi>, "IndOwner"=w217:refnum<vi>, "SourcePosition"=w216:T1, "BundlerIndex"=w204:i32)
        n86 = Multiply(x=w204, y=T1 {"Left"=0, "Top"=16}) -> (x*y=w202:T1)
        n87 = Add(x=w216, y=T1 {"Left"=16, "Top"=24}) -> (x+y=w206:T1)
        n88 = Add(x=w206, y=w202) -> (x+y=w205:T1)
        n89 = New VI Object(vi object class=refnum<vi> refnum ("Bundler"), owner refnum=w217, position/next to=w205, 6:w214, 8:w218) -> (object refnum=w219:refnum<vi>, 0:w220:errorcluster)  [unwired: 3 in]
        n90 = property class="SubVI"(reference=w219, error in=w220, "Position"=w205) -> (reference out=w192:refnum<vi>, error out=w211:errorcluster, "Terms[]"=w194:refnum<vi>[])
        n91 = call <resource>:"Scripting_IndicateConnectorPaneCorners.vi"("Terminals[]"=w194) -> ("RightTop"=w212:i32, "LeftTop"=w213:i32)  [unwired: 7 in, 2 out]
        n92 = Index Array(array=w194, index #1=w213, index #2=w212) -> (element #1=w198:refnum<vi>, element #2=w196:refnum<vi>)
        n93 = Not A Number/Path/Refnum?(number/path/refnum=w194) -> (NaN/Path/Refnum?=w193:bool[])
        n94 = Not A Number/Path/Refnum?(number/path/refnum=w198) -> (NaN/Path/Refnum?=w197:bool)
        n95 = case shown="False" w197 {
          tunnel: w211 -> [w230 w231]
          tunnel: w210 -> [w229 _]
          tunnel: [w228 w231] -> w209
          tunnel: w198 -> [w227 _]
          tunnel: w193 -> [_ _]
          frame False {
            n96 = invoke class="Term" method="Connect Wire"(reference=w227, error in=w230, "Wire Source"=w229) -> (error out=w228:errorcluster)  [unwired: 4 in, 6 out]
          }
          frame True {
          }
        }
        n97 = Not A Number/Path/Refnum?(number/path/refnum=w196) -> (NaN/Path/Refnum?=w195:bool)
        n98 = case shown="False" w195 {
          tunnel: w209 -> [w225 w226]
          tunnel: w208 -> [w224 _]
          tunnel: [w223 w226] -> w207
          tunnel: w196 -> [w222 _]
          frame False {
            n99 = invoke class="Term" method="Connect Wire"(reference=w222, error in=w225, "Wire Source"=w224) -> (error out=w223:errorcluster)  [unwired: 4 in, 6 out]
          }
          frame True {
          }
        }
        n100 = Close Reference(reference=w194, error in (no error)=w207) -> (error out=w201:errorcluster)
        n101 = Close Reference(reference=w192, error in (no error)=w201) -> ()  [unwired: 1 out]
      }
    }
    n102 = Equal?(x=w20, y="Exit") -> (x = y?=w23:bool)
    n103 = Select(t="Error", s=w19, f=w20) -> (s? t:f=w24:string)
  }
  "error out" <- w8
